vi "Set and Get Num of Rows.vi"(7 "Mode":T1, 8 "错误输入":errorcluster, 10 "Number of Rows In":u32, 11 "Listbox Ref":refnum<vi>) -> (0 "错误输出":errorcluster, 2 "Number of Rows Out":u32, 3 "Dup Listbox Ref":refnum<vi>)   [LabVIEW 2011, in "Listbox Tool.lvlib"]
uses:
  Listbox Tool.lvlib
  Custom Type/Read and Write Mode.ctl
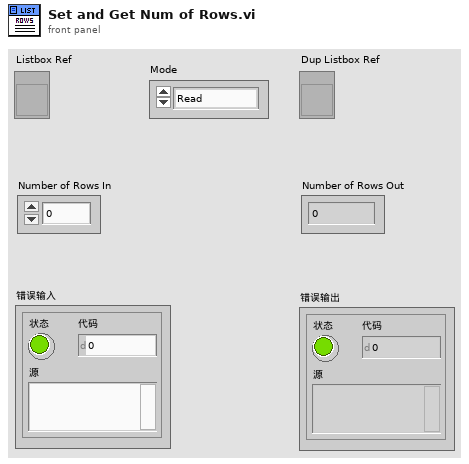
[diagram p1: front panel]
types:
  T1 = typedef "Listbox Tool.lvlib/Read and Write Mode.ctl" = enum16{"Read", "Write"}
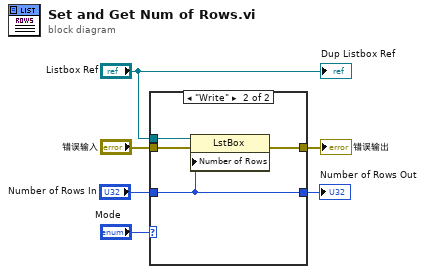
[diagram p0: block diagram]
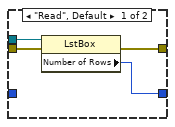
[diagram p2: hidden frame]
diagram:
  n1 = case shown="\"Write\"" "Mode" {
    tunnel: "Listbox Ref" -> [w9 w14]
    tunnel: [w8 w11] -> w2
    tunnel: "错误输入" -> [w10 w13]
    tunnel: [w7 w12] -> w4
    tunnel: "Number of Rows In" -> [_ w11]
    frame "Read", Default {
      n2 = property class="LstBox"(reference=w9, error in=w10) -> (error out=w7:errorcluster, "Number of Rows"=w8:u32)  [unwired: 1 out]
    }
    frame "Write" {
      n3 = property class="LstBox"(reference=w14, error in=w13, "Number of Rows"=w11) -> (error out=w12:errorcluster)  [unwired: 1 out]
    }
  }
  "错误输出" <- w4
  "Number of Rows Out" <- w2
  "Dup Listbox Ref" <- "Listbox Ref"
